vi "FP_Move to Point.vi"(7 "Target Point":T1, 8 "Error":errorcluster, 9 "FP Position":T2, 11 "VI":refnum<vi>) -> (0 "Error Out":errorcluster, 3 "VI Out":refnum<vi>)   [LabVIEW 2016]
uses:
  TypeDefs_Utility/ENUM RB_Pos_Quadrant Position.ctl
  TypeDefs_Utility/Cluster_Pos_Top Left position.ctl
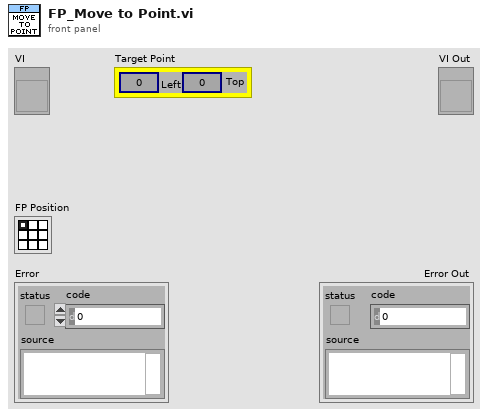
[diagram p1: front panel]
types:
  T1 = typedef "Cluster_Pos_Top Left position.ctl" = cluster{"Left":i16, "Top":i16}
  T2 = typedef "ENUM RB_Pos_Quadrant Position.ctl" = enum32{"LFT-TOP", "MID-TOP", "RGT-TOP", "LFT-CTR", "MID-CTR", "RGT-CTR", "LFT-BOT", "MID-BOT", "RGT-BOT"}
  T3 = typedef "LVRectTypeDef.ctl" = cluster{"Left":i16, "Top":i16, "Right":i16, "Bottom":i16}
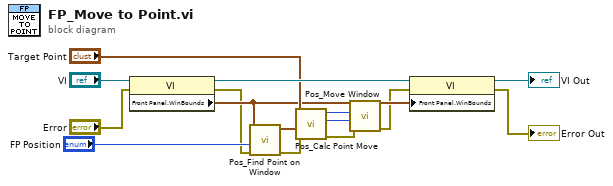
[diagram p0: block diagram]
diagram:
  n1 = property class="VI"(reference="VI", error in="Error") -> (reference out=w15:refnum<vi>, error out=w4:errorcluster, "Front Panel.WinBounds"=w5:T3)
  n2 = call "Pos_Find Point on Window.vi"("Error"=w4, "Position"="FP Position", "Window"=w5) -> ("Error Out"=w3:errorcluster, "Point Out"=w11:T1)  [unwired: 7 in]
  n3 = call "Pos_Calc Point Move.vi"("Error"=w3, "Current Location"=w11, "Tartget Location"="Target Point") -> ("Error Out"=w2:errorcluster, "Down Out"=w10:i16, "Right Out"=w9:i16)  [unwired: 6 in]
  n4 = call "Pos_Move Window.vi"("Error"=w2, "Down"=w10, "Right"=w9, "Window"=w5) -> ("Error Out"=w1:errorcluster, "Window Out"=w7:T3)  [unwired: 6 in]
  n5 = property class="VI"(reference=w15, error in=w1, "Front Panel.WinBounds"=w7) -> (reference out=→"VI Out":refnum<vi>, error out=→"Error Out":errorcluster)
